vi "S2C_ProcessFGV.vi"(8 "Error In":errorcluster, 10 "Q-Ref":refnum<queue>, 11 "Action":enum16{"Init", "Add", "Get"}(ring)) -> (0 "Error Out":errorcluster, 3 "Q-Array":refnum<queue>[](array[refnum]))   [LabVIEW 2024]
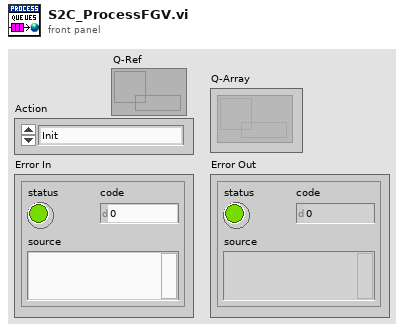
[diagram p1: front panel]
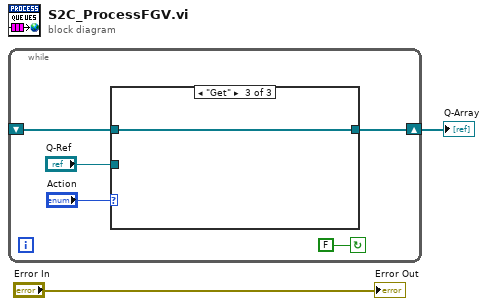
[diagram p0: block diagram]
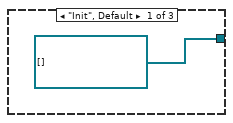
[diagram p2: hidden frame]
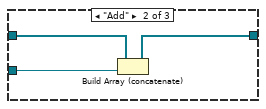
[diagram p3: hidden frame]
diagram:
  n1 = while {
    shift-right: [w5] -> w1
    shift-left: _ -> [w4]
    stop <- FALSE continue-if-true
    n2 = case shown="\"Get\"" "Action" {
      tunnel: [refnum<queue>[] [] ("Q-Array") w10 w12] -> w5
      tunnel: w4 -> [_ w11 w12]
      tunnel: "Q-Ref" -> [_ w9 _]
      frame "Init", Default {
      }
      frame "Add" {
        n3 = Build Array (concatenate)(w11, w9) -> (w10:refnum<queue>[])
      }
      frame "Get" {
      }
    }
  }
  "Q-Array" <- w1
  "Error Out" <- "Error In"
